vi "Do.vi"(8 "error in (no error)":errorcluster, 10 "Actor in":refnum<class "Actor.lvclass">, 11 "Cooler Update Water Level Msg":refnum<class "Cooler Update Water Level Msg.lvclass">) -> (0 "error out":errorcluster, 2 "Actor out":refnum<class "Actor.lvclass">)   [LabVIEW 2025, in "Evaporative Cooler.lvlib" / "Cooler Update Water Level Msg.lvclass"]
uses:
  Cooler Update Water Level Msg.lvclass
  <vilib>/ActorFramework/Actor/Actor.lvclass
  Evaporative Cooler/Evaporative Cooler.lvclass
  Water Level/Update Water Level Msg/Update Water Level Msg.lvclass/Update Water Level Msg.ctl
  Water Level/Update Water Level Msg/Update Water Level Msg.lvclass
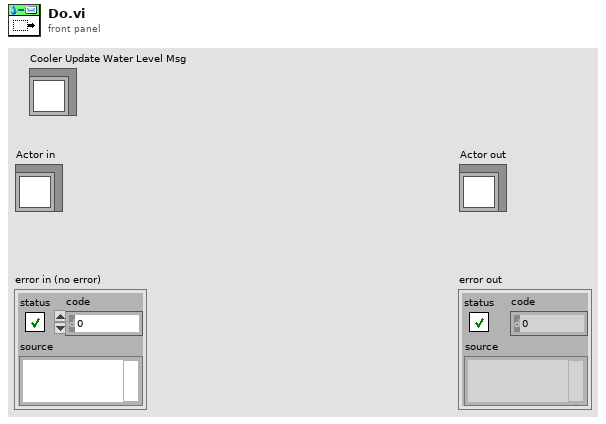
[diagram p1: front panel]
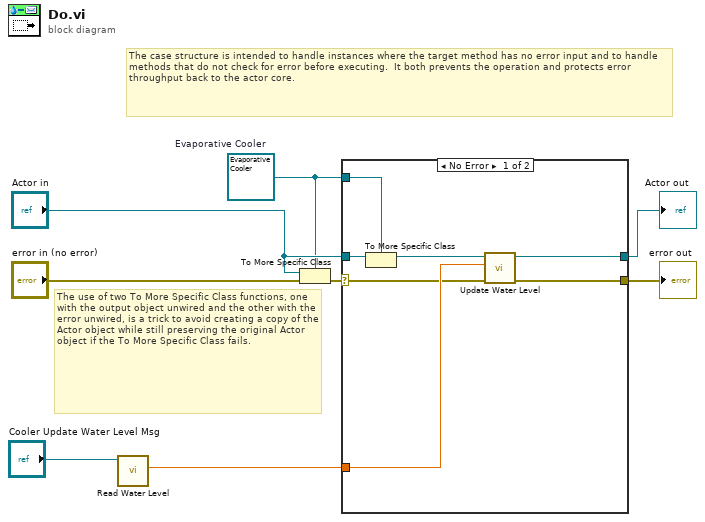
[diagram p0: block diagram]
diagram:
  w1 = refnum<class "Evaporative Cooler.lvclass"> refnum  # Evaporative Cooler
  # "The use of two To More Specific Class functions, one with the output object unwired and the other with the error unwired, is a trick to avoid creating a copy of the Actor object while still preserving the original Actor object if the To More Specific Class fails."
  # "The case structure is intended to handle instances where the target method has no error input and to handle methods that do not check for error before executing.  It both prevents the operation and protects error throughput back to the actor core."
  n1 = call "Read Water Level.vi"("Update Water Level Msg in"="Cooler Update Water Level Msg") -> ("Water Level"=w2:dbl)  [unwired: 9 in, 1 out]
  n2 = To More Specific Class(target class=w1, reference="Actor in", error in="error in (no error)") -> (error out=w7:errorcluster)  [unwired: 1 out]
  n3 = case shown="No Error" w7 {
    selector: w7 -> [w9 w17]
    tunnel: [w11 w17] -> w6
    tunnel: [w12 w16] -> w5
    tunnel: "Actor in" -> [w15 w16]
    tunnel: w1 -> [w14 _]
    tunnel: w2 -> [w10 _]
    frame No Error {
      n4 = To More Specific Class(target class=w14, reference=w15) -> (specific class reference=w13:refnum<class "Evaporative Cooler.lvclass">)  [unwired: 1 in, 1 out]
      n5 = call "Update Water Level.vi"("error in (no error)"=w9, "Water Level"=w10, "Evaporative Cooler"=w13) -> ("error out"=w11:errorcluster, "Evaporative Cooler"=w12:refnum<class "Evaporative Cooler.lvclass">)  [unwired: 7 in]
    }
    frame Error {
      # "If type check fails, pass the original object out again."
    }
  }
  "error out" <- w6
  "Actor out" <- w5
